vi "Descend.vi"(8 "error in (no error)":errorcluster, 10 "Path Tokens":string[](array[string]), 11 "PathTreeNode in":refnum<class "PathTreeNode.lvclass">) -> (0 "error out":errorcluster, 1 "Child Token":string, 2 "Remaining Tokens":string[](array[string]), 3 "PathTreeNode out":refnum<class "PathTreeNode.lvclass">)   [LabVIEW 2020, in "PathTree.lvlib" / "PathTreeNode.lvclass"]
uses:
  PathTreeNode.lvclass
  PathTreeNode.lvclass/PathTreeNode.ctl
  <vilib>/Utility/error.llb/Error Cluster From Error Code.vi
  <vilib>/ErrorRing/Error Ring.xnode
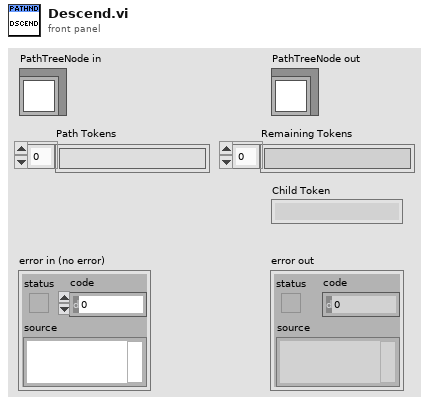
[diagram p1: front panel]
types:
  T1 = typedef "Advanced Structures.lvlib/PathTreeNode.lvclass/Ref Data.ctl" = cluster{"Tree":refnum<class>, "Parent":refnum<class>, "Token":string, "Child Tokens":string[], "Child Nodes":refnum<class>[], "Value":refnum<class>, "Has Value":bool}
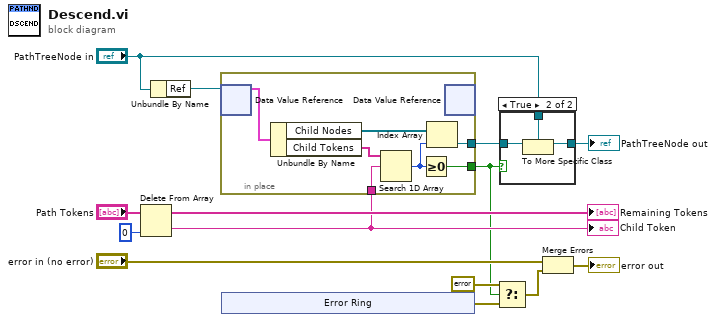
[diagram p0: block diagram]
diagram:
  n1 = Delete From Array(array="Path Tokens", index=0) -> (deleted portion=w10:string, array with subset deleted=→"Remaining Tokens":string[])  [unwired: 1 in]
  "Child Token" <- w10
  n2 = Unbundle By Name("PathTreeNode in") -> ("Ref"=w11:refnum<data-value>)
  n3 = in-place {
    in-place-border: w10 -> [w19]
    in-place-border: [w16] -> w4
    in-place-border: [w15] -> w5
    n4 = in-place-dvr #1(w11) -> (w21:T1)  [unwired: 1 out]
    n5 = Unbundle By Name(w21) -> ("Child Nodes"=w18:refnum<class>[], "Child Tokens"=w20:string[])
    n6 = Search 1D Array(1D array=w20, element=w19) -> (index of element=w17:i32)  [unwired: 1 in]
    n7 = Greater Or Equal To 0?(x=w17) -> (x >= 0?=w15:bool)
    n8 = Index Array(array=w18, index=w17) -> (element=w16:refnum<class>)
    n9 = in-place-dvr #1() -> ()  [unwired: 1 in, 2 out]
  }
  n10 = xnode "Error Ring"() -> ("error out"=w9:errorcluster)
  n11 = Select(t=errorcluster {"status"=FALSE, "code"=0, "source"=""}, s=w5, f=w9) -> (s? t:f=w6:errorcluster)
  n12 = case shown="True" w5 {
    tunnel: w4 -> [_ w25]
    tunnel: "PathTreeNode in" -> [w22 w24]
    tunnel: [w22 w23] -> w2
    frame False {
    }
    frame True {
      n13 = To More Specific Class(target class=w24, reference=w25) -> (specific class reference=w23:refnum<class "PathTreeNode.lvclass">)  [unwired: 1 in, 1 out]
    }
  }
  "PathTreeNode out" <- w2
  n14 = Merge Errors("error in (no error)", w6) -> (→"error out":errorcluster)
